vi "Untitled 1.vi"() -> ()   [LabVIEW 2020]
panel:
  out "error out":errorcluster
  out "function name":string[](array[string])
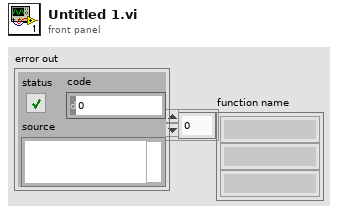
[diagram p1: front panel]
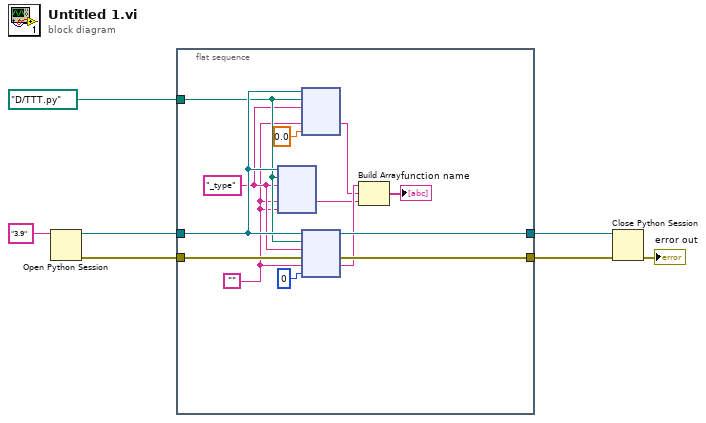
[diagram p0: block diagram]
diagram:
  n1 = Open Python Session(python version="3.9" ("Python version")) -> (session out=w2:refnum<k35>, error out=w7:errorcluster)  [unwired: 2 in]
  n2 = flat-sequence {
    tunnel: w7 -> [w20]
    tunnel: [w19] -> w6
    tunnel: [w18] -> w5
    tunnel: w2 -> [w16]
    tunnel: path "D:/TTT.py" ("module path") -> [w15]
    frame #0 {
      w12 = "" ("function name")
      w14 = "_type" ("function name")
      n3 = node(w16, w15, w14, w12, w12) -> (w9:string)  [unwired: 2 in, 4 out]
      n4 = node(w16, w15, w14, w12, 0.0 ("Numeric")) -> (w10:string)  [unwired: 2 in, 4 out]
      n5 = node(w16, w15, w14, w20, w12, 0 ("Numeric")) -> (w19:refnum<k35>, w18:errorcluster, w11:string)  [unwired: 1 in, 2 out]
      n6 = Build Array(w11, w10, w9) -> (→"function name":string[])
    }
  }
  n7 = Close Python Session(session in=w6, error in=w5) -> (11:→"error out":errorcluster)
